vi "Global_SEN Write_Data.vi"() -> ()   [LabVIEW 2016, in "TemplateSensor.lvlib"]
uses:
  TemplateSensor.lvlib
panel:
  in  "TemplateSensor_SEN_INT":i32
  in  "TemplateSensor_SEN_Bool":bool
  in  "TemplateSensor_SEN_DBL":dbl
  # "The Names of the Data items in the Global Variable MUST describe who the Single Writer is\nNaming Convention of all Data Items is:   \nLib Name_Loop Name (SM or SEN or ACT)_Data Name\nExamples:\nDrive_ACT_X axis\nGameController_SEN_JoystickLeft\nHopper_SM_AgitatorSpeed"
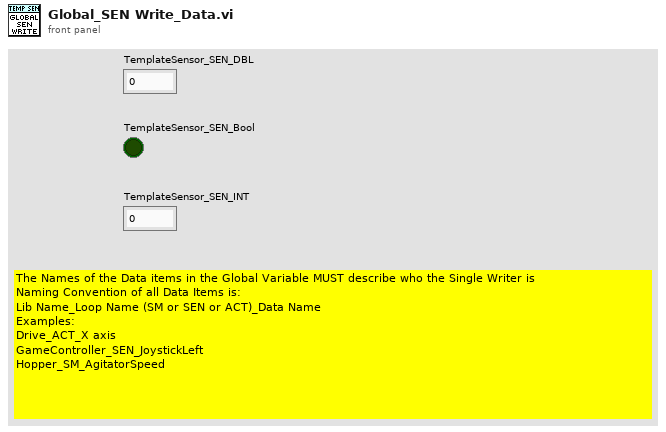
[diagram p1: front panel]
diagram:
